vi "Create Output Sessions.vi"(0 "XNET Output Signal Names":string[](array[string]), 5 "XNET Interface":refnum<k21>, 9 "Num of Signals Per Frame":i32[](array[numeric]), 11 "error in":errorcluster) -> (4 "Output Sessions":refnum<k21>[](array[refnum]), 15 "error out":errorcluster)   [LabVIEW 2009, in "NI-XNET Custom Device.lvlib"]
doc: "This uses creates an array of NI-XNET single-point output sessions according the list of output signals. It creates a seperate output session for each \"frame\", so it need to know how many signals are assigned to each frame."
uses:
  NI-XNET Custom Device.lvlib
  <vilib>/xnet/xnet.llb/XNET Create Session (Signal Output Single-point).vi
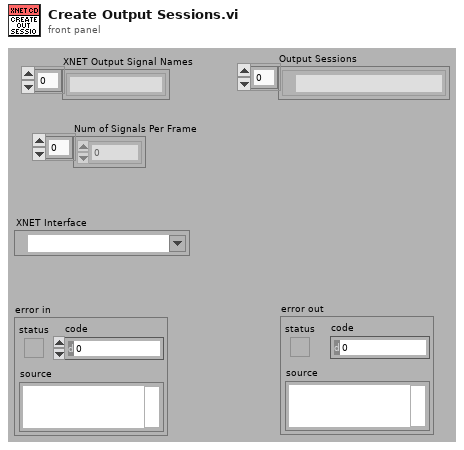
[diagram p1: front panel]
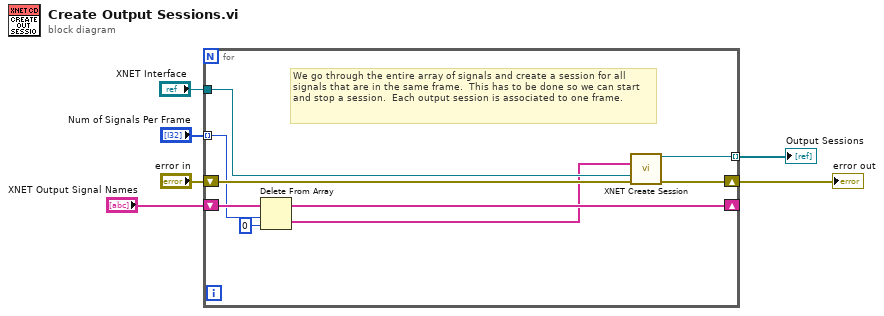
[diagram p0: block diagram]
diagram:
  n1 = for {
    tunnel: "Num of Signals Per Frame" -> [w10] mode=indexing
    tunnel: "XNET Interface" -> [w15]
    shift-right: [w14] -> w4
    shift-left: "error in" -> [w13]
    tunnel: [w12] -> w5 mode=indexing
    shift-right: [w9] -> _
    shift-left: "XNET Output Signal Names" -> [w11]
    # "We go through the entire array of signals and create a session for all signals that are in the same frame.  This has to be done so we can start and stop a session.  Each output session is associated to one frame."
    n2 = Delete From Array(array=w11, length=w10, index=0) -> (deleted portion=w8:string[], array with subset deleted=w9:string[])
    n3 = call-poly <vilib>:"XNET Create Session.vi"("signal list"=w8, "interface"=w15, "error in (no error)"=w13) -> ("session out"=w12:refnum<k21>, "error out"=w14:errorcluster)  [unwired: 11 in]
  }
  "Output Sessions" <- w5
  "error out" <- w4
